vi "Check Action.vi"(6 "HRS Time":dbl, 7 "Values In":dbl[](array[numeric]), 8 "error in (no error)":errorcluster, 11 "SequencedValves in":refnum<class "TriggerDelayControl.lvclass">) -> (0 "error out":errorcluster, 1 "Do Action":bool, 2 "Action":T1, 3 "SequencedValves out":refnum<class "TriggerDelayControl.lvclass">, 5 "Values":dbl[](array[numeric]))   [LabVIEW 2020, in "VolatusControl.lvlib" / "TriggerDelayControl.lvclass"]
uses:
  TriggerDelayControl.lvclass
  TriggerDelayControl.lvclass/TriggerDelayControl.ctl
  Volatus/MessageQ/MessageQ.lvclass
  Valve Action.ctl
  VolatusControl.lvlib
  State.ctl
  lv-vecto/Vecto/Channel/Channel.lvclass
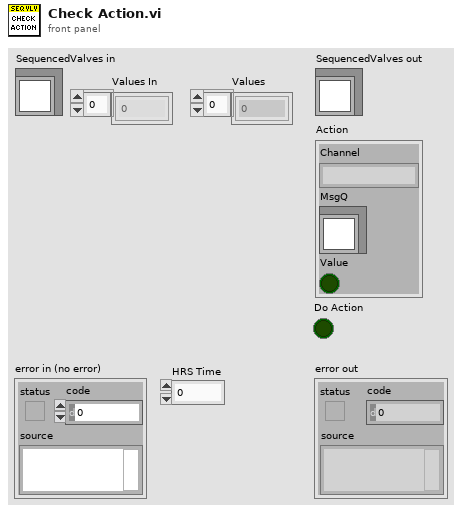
[diagram p1: front panel]
types:
  T1 = typedef "VolatusControl.lvlib/Valve Action.ctl" = cluster{"Channel":string, "MsgQ":refnum<class "MessageQ.lvclass">, "Value":bool}
  T2 = typedef "VolatusControl.lvlib/TriggerDelayControl.lvclass/State.ctl" = enum16{"Idle", "Start", "Trigger", "Delay"}
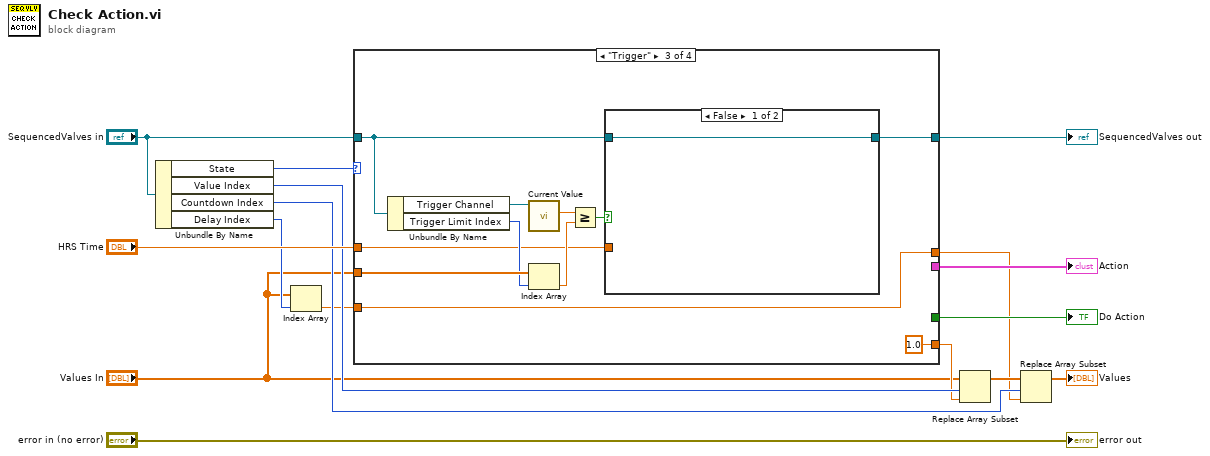
[diagram p0: block diagram]
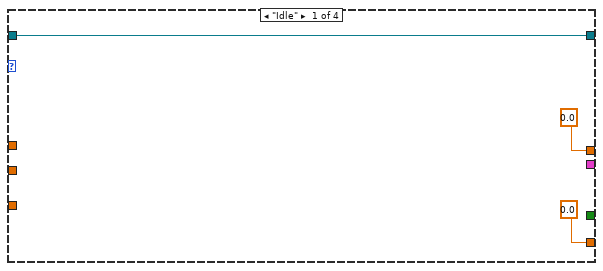
[diagram p2: hidden frame]
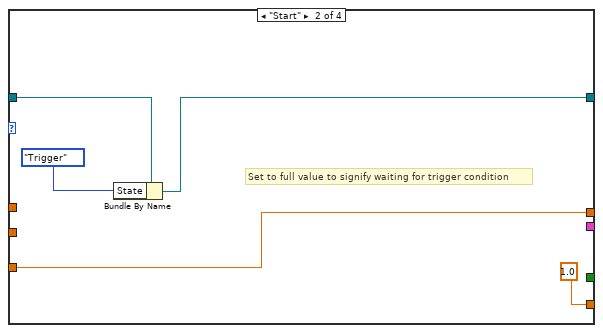
[diagram p3: hidden frame]
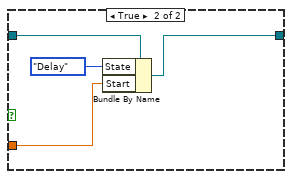
[diagram p4: hidden frame]
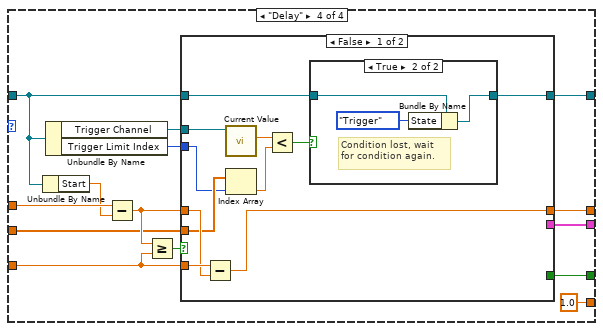
[diagram p5: hidden frame]
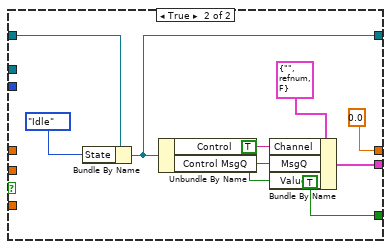
[diagram p7: hidden frame]
diagram:
  n1 = Unbundle By Name("SequencedValves in") -> ("State"=w15:T2, "Value Index"=w9:i32, "Countdown Index"=w6:i32, "Delay Index"=w4:i32)
  n2 = Index Array(array="Values In", index=w4) -> (element=w5:dbl)
  n3 = case shown="\"Trigger\"" w15 {
    tunnel: "SequencedValves in" -> [w19 w24 w28 w44]
    tunnel: "HRS Time" -> [_ _ w27 w54]
    tunnel: [w19 w22 w26 w51] -> w12
    tunnel: [_ _ _ w50] -> w11
    tunnel: [_ _ _ w49] -> w10
    tunnel: [0.0 1.0 1.0 1.0] -> w8
    tunnel: w5 -> [_ w20 w35 w45]
    tunnel: [0.0 ("Numeric") w20 w35 w46] -> w3
    tunnel: "Values In" -> [_ _ w34 w43]
    frame "Idle" {
    }
    frame "Start" {
      # "Set to full value to signify waiting for trigger condition"
      n4 = Bundle By Name(cluster=w24, "State"=State."Trigger") -> (w22:refnum<class "TriggerDelayControl.lvclass">)
    }
    frame "Trigger" {
      n5 = Unbundle By Name(w28) -> ("Trigger Channel"=w32:refnum<class "Channel.lvclass">, "Trigger Limit Index"=w33:i32)
      n6 = call "Current Value.vi"("Channel in"=w32) -> ("Scaled"=w31:dbl)  [unwired: 6 in, 4 out]
      n7 = Index Array(array=w34, index=w33) -> (element=w30:dbl)
      n8 = Greater Or Equal?(x=w31, y=w30) -> (x >= y?=w29:bool)
      n9 = case shown="False" w29 {
        tunnel: w28 -> [w36 w40]
        tunnel: w27 -> [_ w38]
        tunnel: [w36 w37] -> w26
        frame False {
        }
        frame True {
          n10 = Bundle By Name(cluster=w40, "State"=State."Delay", "Start"=w38) -> (w37:refnum<class "TriggerDelayControl.lvclass">)
        }
      }
    }
    frame "Delay" {
      n11 = Unbundle By Name(w44) -> ("Start"=w53:dbl)
      n12 = Unbundle By Name(w44) -> ("Trigger Channel"=w42:refnum<class "Channel.lvclass">, "Trigger Limit Index"=w41:i32)
      n13 = Subtract(x=w54, y=w53) -> (x-y=w47:dbl)
      n14 = Greater Or Equal?(x=w47, y=w45) -> (x >= y?=w52:bool)
      n15 = case shown="False" w52 {
        tunnel: w44 -> [w57 w74]
        tunnel: [w55 w73] -> w51
        tunnel: [_ w76] -> w50
        tunnel: [_ TRUE] -> w49
        tunnel: w47 -> [w64 _]
        tunnel: [w63 0.0] -> w46
        tunnel: w45 -> [w65 _]
        tunnel: w43 -> [w60 _]
        tunnel: w42 -> [w61 _]
        tunnel: w41 -> [w59 _]
        frame False {
          n16 = Subtract(x=w65, y=w64) -> (x-y=w63:dbl)
          n17 = call "Current Value.vi"("Channel in"=w61) -> ("Scaled"=w62:dbl)  [unwired: 6 in, 4 out]
          n18 = Index Array(array=w60, index=w59) -> (element=w58:dbl)
          n19 = Less?(x=w62, y=w58) -> (x < y?=w56:bool)
          n20 = case shown="True" w56 {
            tunnel: w57 -> [w66 w69]
            tunnel: [w66 w67] -> w55
            frame False {
            }
            frame True {
              # "Condition lost, wait for condition again."
              n21 = Bundle By Name(cluster=w69, "State"=State."Trigger") -> (w67:refnum<class "TriggerDelayControl.lvclass">)
            }
          }
        }
        frame True {
          n22 = Bundle By Name(cluster=w74, "State"=State."Idle") -> (w73:refnum<class "TriggerDelayControl.lvclass">)
          n23 = Unbundle By Name(w73) -> ("Control"=w71:string, "Control MsgQ"=w77:refnum<class "MessageQ.lvclass">)
          n24 = Bundle By Name(cluster=T1 {"Channel"="", "MsgQ"=refnum, "Value"=FALSE} ("Action"), "Channel"=w71, "MsgQ"=w77, "Value"=TRUE) -> (w76:T1)
        }
      }
    }
  }
  "SequencedValves out" <- w12
  "Action" <- w11
  "Do Action" <- w10
  n25 = Replace Array Subset(array="Values In", new element=w8, index=w9) -> (w7:dbl[])
  n26 = Replace Array Subset(array=w7, new element=w3, index=w6) -> (→"Values":dbl[])
  "error out" <- "error in (no error)"
